vi "题目 3 温度测量子VI.vi"(1 "停止":bool, 3 "温度单位":bool) -> (0 "温度计":dbl(slide) scale=0.0..260.0, 2 "温度":string)   [LabVIEW 2017]
panel:
  # "℉"
  # "℃"
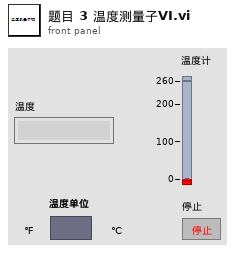
[diagram p1: front panel]
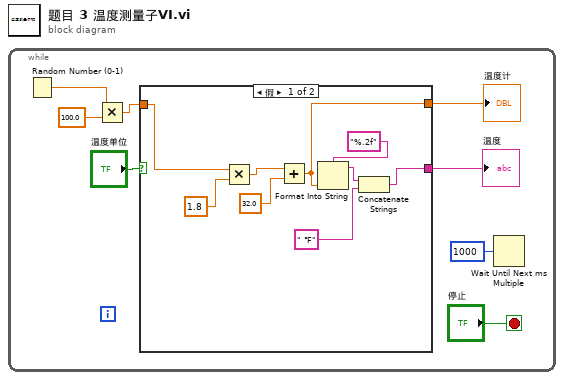
[diagram p0: block diagram]
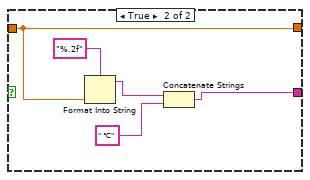
[diagram p2: hidden frame]
diagram:
  n1 = while {
    stop <- "停止" stop-if-true
    n2 = Random Number (0-1)() -> (number: 0 to 1=w7:dbl)
    n3 = Multiply(x=w7, y=100.0) -> (x*y=w4:dbl)
    n4 = case shown="假" "温度单位" {
      tunnel: w4 -> [w17 w19]
      tunnel: [w11 w20] -> w3
      tunnel: [w10 w19] -> w2
      frame False {
        n5 = Multiply(x=w17, y=1.8) -> (x*y=w15:dbl)
        n6 = Add(x=w15, y=32.0) -> (x+y=w10:dbl)
        n7 = Format Into String(format string="%.2f" ("格式字符串"), w10) -> (resulting string=w13:string)  [unwired: 2 in, 1 out]
        n8 = Concatenate Strings(w13, " ℉") -> (w11:string)
      }
      frame True {
        n9 = Format Into String(format string="%.2f" ("格式字符串"), w19) -> (resulting string=w22:string)  [unwired: 2 in, 1 out]
        n10 = Concatenate Strings(w22, " ℃" ("字符串")) -> (w20:string)
      }
    }
    "温度" <- w3
    "温度计" <- w2
    n11 = Wait Until Next ms Multiple(millisecond multiple=u32 1000 ("毫秒倍数")) -> ()  [unwired: 1 out]
  }
